vi "Insert View.vi"(8 "error in (no error)":errorcluster, 9 "Insertion Request Time":timestamp, 10 "Protected Subpanel":refnum<data-value>, 11 "IViewable in":refnum<class "IViewable.lvclass">) -> (0 "error out":errorcluster, 3 "IViewable out":refnum<class "IViewable.lvclass">)   [LabVIEW 2015, in "IViewable.lvlib" / "IViewable.lvclass"]
doc: "<License>\nCopyright © 2017 Composed Systems, LLC | All rights reserved\nwww.composed.io\n\nAuthor: Ethan Stern <ethan.stern@composed.io>\n\nThis software is provided \"AS IS\" WITHOUT WARRANTIES, either express or implied, AND IS FOR EDUCATIONAL PURPOSES ONLY.\n</License>"
uses:
  IViewable.lvclass
  ProtectedSubpanel/ProtectedSubpanel.lvclass
  IViewable.lvclass/IViewable.ctl
  <vilib>/Utility/LVClass/Get LV Class Name.vi
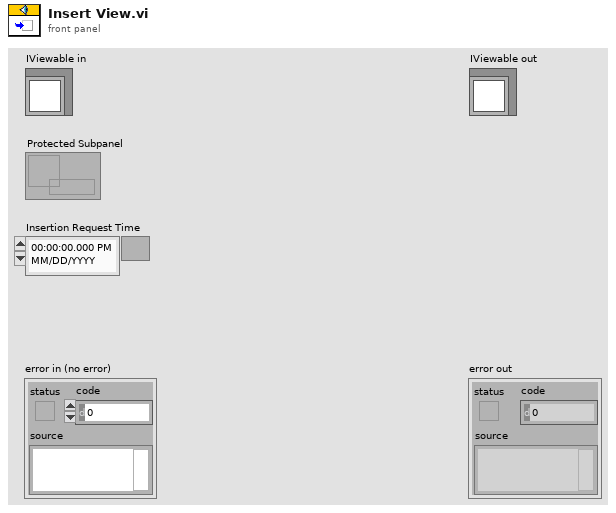
[diagram p1: front panel]
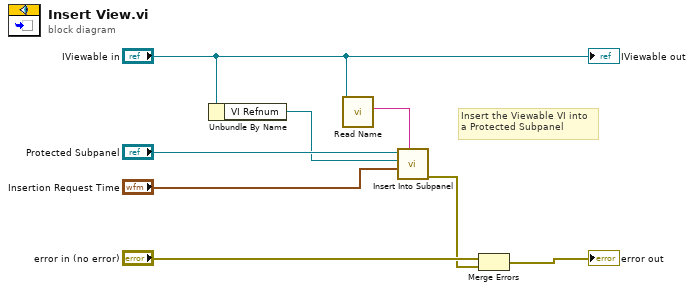
[diagram p0: block diagram]
diagram:
  # "Insert the Viewable VI into\na Protected Subpanel"
  n1 = Unbundle By Name("IViewable in") -> ("VI Refnum"=w5:refnum<vi>)
  n2 = call "Read Name.vi"("IViewable In"="IViewable in") -> ("Name"=w1:string)  [unwired: 8 in, 2 out]
  n3 = call "Insert Into Subpanel.vi"("View Name"=w1, "Insertion Request Time"="Insertion Request Time", "VI Refnum"=w5, "Protected Subpanel"="Protected Subpanel") -> ("error out"=w3:errorcluster)  [unwired: 6 in, 1 out]
  n4 = Merge Errors("error in (no error)", w3) -> (→"error out":errorcluster)
  "IViewable out" <- "IViewable in"
